vi "Set Board ID.vi"(8 "error in":errorcluster, 10 "Board ID":i32, 11 "custom device ref":T1 format="%.0x") -> (0 "error out":errorcluster, 3 "custom device ref out":T1 format="%.0x")   [LabVIEW 2020, in "AIM ARINC 664 Scripting.lvlib"]
uses:
  AIM ARINC 664 Scripting.lvlib
  <vilib>/NI VeriStand/Custom Device API/Custom Device Item Ref.ctl
  Constants.vi
  <vilib>/NI VeriStand/Custom Device API/Custom Device API.lvlib
  <vilib>/NI VeriStand/Custom Device API/Set Item Property (I32).vi
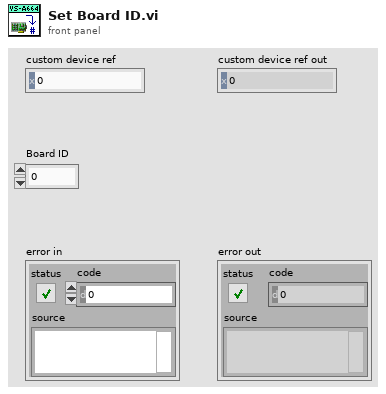
[diagram p1: front panel]
types:
  T1 = typedef "Custom Device API.lvlib/Custom Device Item Ref.ctl" = u64
  T2 = typedef "AIM ARINC 664 Import.lvlib/board_setup.ctl" = cluster{"boardId":u32, "portSpeed":u32, "portConfig":u32}
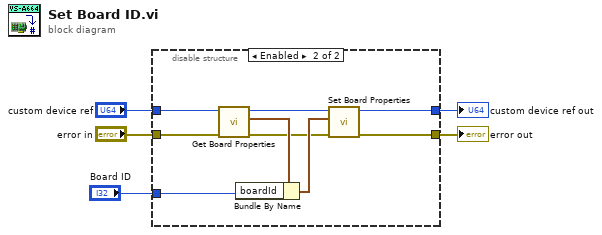
[diagram p0: block diagram]
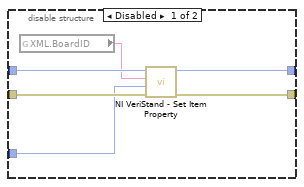
[diagram p2: hidden frame]
diagram:
  n1 = disable-structure shown="Enabled" {
    disable-tunnel: "custom device ref" -> [w11 w20]
    disable-tunnel: "error in" -> [w10 w19]
    disable-tunnel: [w9 w12] -> w3
    disable-tunnel: [w8 w13] -> w2
    disable-tunnel: "Board ID" -> [w7 w17]
    frame Disabled {
      n2 = global read "Constants.vi" "XML.BoardID"() -> (w6:string)
      n3 = call-poly <vilib>:"NI VeriStand - Set Item Property.vi"("error in (no error)"=w10, "Value"=w7, "Property Name"=w6, "Item Ref in"=w11) -> ("error out"=w8:errorcluster, "Item Ref out"=w9:T1)  [unwired: 5 in, 1 out]
    }
    frame Enabled {
      n4 = call "Get Board Properties.vi"("error in"=w19, "custom device ref"=w20) -> ("error out"=w14:errorcluster, "board properties out"=w18:T2, "custom device ref out"=w15:T1)  [unwired: 7 in]
      n5 = Bundle By Name(cluster=w18, "boardId"=w17) -> (w16:T2)
      n6 = call "Set Board Properties.vi"("error in"=w14, "board setup"=w16, "custom device ref in"=w15) -> ("error out"=w13:errorcluster, "custom device ref out"=w12:T1)  [unwired: 6 in, 1 out]
    }
  }
  "custom device ref out" <- w3
  "error out" <- w2
